vi "Read DTCs.vi"(8 "error in (no error)":errorcluster, 11 "Node Ptr":T2 format="%.0x") -> (0 "error out":errorcluster)   [LabVIEW 2024, in "Diagnostics Addon System Explorer.lvlib"]
uses:
  Diagnostics Addon System Explorer.lvlib
  <vilib>/NI VeriStand/Custom Device API/Custom Device Item Ref.ctl
  Types/FG.Action.ctl
  Addon Shared/Types/DTC.Settings.ctl
  Addon Shared/Types/DTC.Descriptor.ctl
  <vilib>/NI VeriStand/Custom Device API/Custom Device Channel.ctl
  <vilib>/NI VeriStand/Custom Device API/Custom Device Channel Type.ctl
  Addon Shared/SubVIs/Constants.vi
  <vilib>/NI VeriStand/Custom Device Tools/Custom Device Utility Library/NI VeriStand - Search for All Items by GUID.vi
  <vilib>/NI/NI VeriStand Advanced SysDef API/SysDef API/SysDef.Property.Set.vi
  <vilib>/NI/NI VeriStand Advanced SysDef API/_SubVIs/SysDef.Property.Set.I32.vi
  <vilib>/NI/NI VeriStand Advanced SysDef API/_SubVIs/SysDef.Property.Set.U32.vi
  <vilib>/NI/NI VeriStand Advanced SysDef API/_SubVIs/SysDef.Property.Set.DBL.Array.vi
  <vilib>/NI/NI VeriStand Advanced SysDef API/_SubVIs/SysDef.Property.Set.String.Array.vi
  <vilib>/NI VeriStand/Custom Device API/NI VeriStand - Get Item Property.vi
  <vilib>/NI VeriStand/Custom Device API/Get Item Property (I32).vi
  <vilib>/NI VeriStand/Custom Device API/Get Item Property (U32).vi
  <vilib>/NI VeriStand/Custom Device API/Get Item Property (Double Array).vi
  <vilib>/NI VeriStand/Custom Device API/Get Item Property (String Array).vi
  <vilib>/NI VeriStand/Custom Device Tools/Custom Device Utility Library/NI VeriStand - Search for Item by GUID.vi
  <vilib>/NI VeriStand/Custom Device API/Custom Device API.lvlib
  Addon Shared/Diagnostics Addon Shared.lvlib
  <vilib>/NI VeriStand/Custom Device Tools/Custom Device Utility Library/Custom Device Utility Library.lvlib
panel:
  in  "Clear":bool
  in  "Code Tabs":T1(tab)
  in  "DTC Byte Length":i32=2
  in  "Status Byte Length":i32=1
  in  "Failure Byte Length":i32=1
  in  "Byte Order":enum16{"Motorola", "Intel"}(ring)
  in  "DTC Codes":i32(listbox)
  in  "Status Codes":i32(listbox)
  in  "Import":bool
  in  "Apply":bool
  in  "Number of DTCs":u32=10 min=1 step=1
  in  "Header 2":cluster{"Section Name":string}={"Section Name"="Number of DTCs to Acquire"}
  in  "Description":string
  out "Name":string
  in  "SHDocVw.IWebBrowser":refnum<k7>(container)
  in  "Header":cluster{"Section Name":string}={"Section Name"="DTC Settings"}
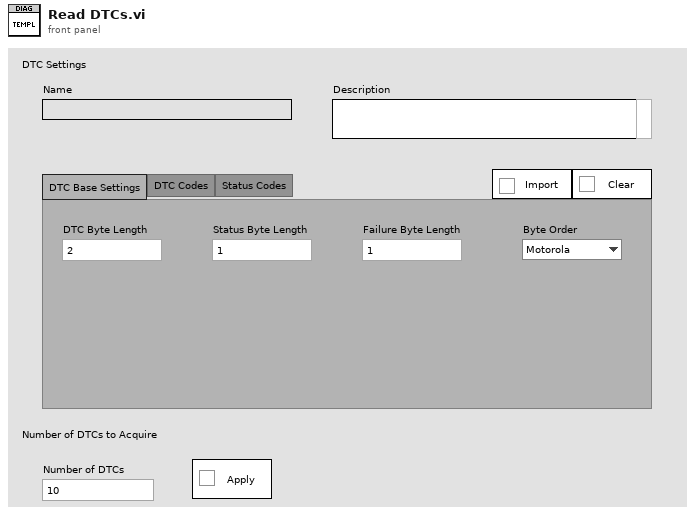
[diagram p1: front panel]
types:
  T1 = enum32{"DTC Base Settings", "DTC Codes", "Status Codes"}
  T2 = typedef "Custom Device API.lvlib/Custom Device Item Ref.ctl" = u64
  T3 = typedef "Diagnostics Addon Shared.lvlib/DTC.Settings.ctl" = cluster{"Descriptor":T4, "Value.Code":dbl[], "Value.String":string[], "Value.J2012String":string[], "Status.Code":dbl[], "Status.String":string[]}
  T4 = typedef "Diagnostics Addon Shared.lvlib/DTC.Descriptor.ctl" = cluster{"DTC Byte Length":i32, "Status Byte Length":i32, "Add Data Byte Length":i32, "Byte Order":enum16{"Motorola", "Intel"}}
  T5 = typedef "Diagnostics Addon System Explorer.lvlib/FG.Action.ctl" = enum16{"Get", "Set"}
  T6 = typedef "Custom Device API.lvlib/Custom Device Item Info.ctl" = cluster{"Name":string, "Is Channel":bool, "GUID":string, "Is Waveform":bool}
  T7 = typedef "Custom Device API.lvlib/Custom Device Channel.ctl" = cluster{"Type":T8, "Units":string, "Default Value":dbl, "Faultable":bool, "Scalable":bool}
  T8 = typedef "Custom Device API.lvlib/Custom Device Channel Type.ctl" = enum16{"Input", "Output"}
  T9 = typedef "Custom Device API.lvlib/Custom Device Commands.ctl" = enum16{"Default", "Item renamed", "Shutdown", "Dynamic button pressed"}
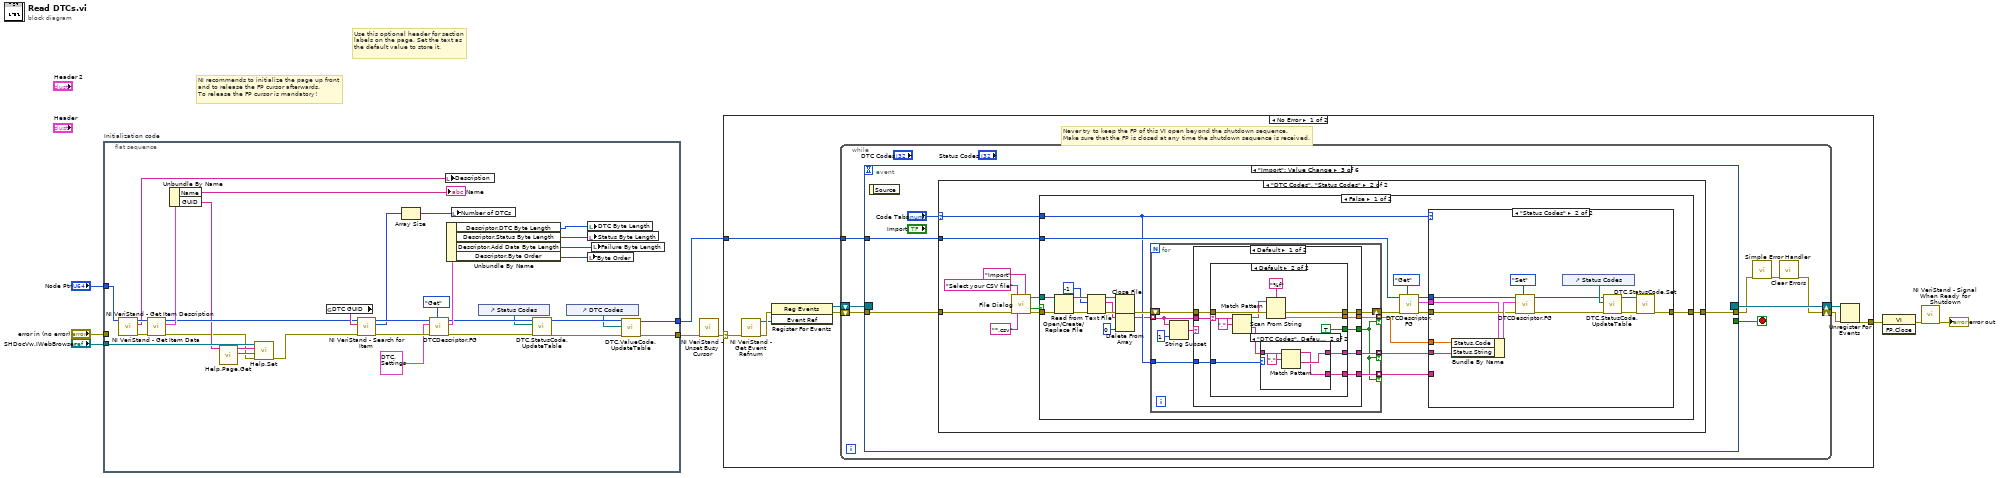
[diagram p0: block diagram]
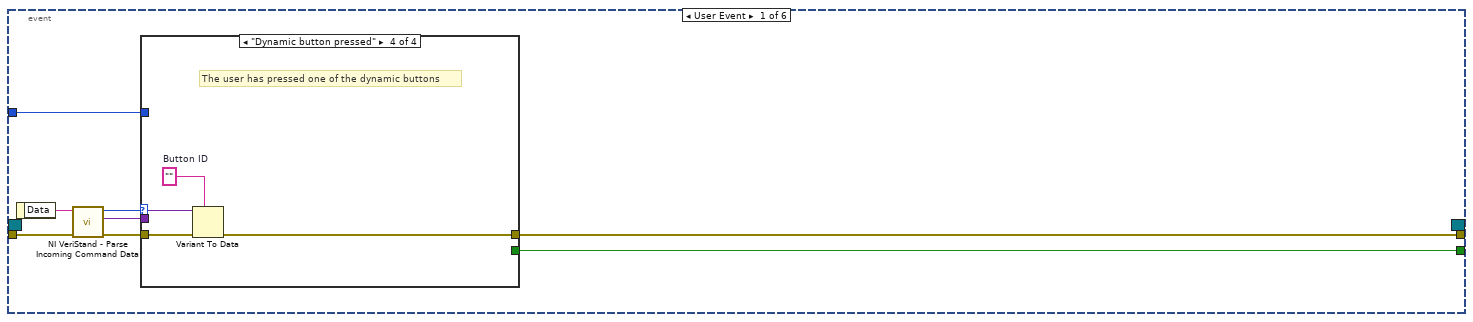
[diagram p2: hidden frame]
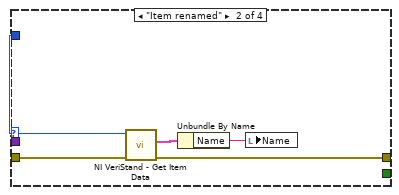
[diagram p4: hidden frame]
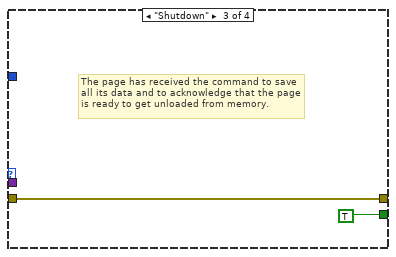
[diagram p5: hidden frame]
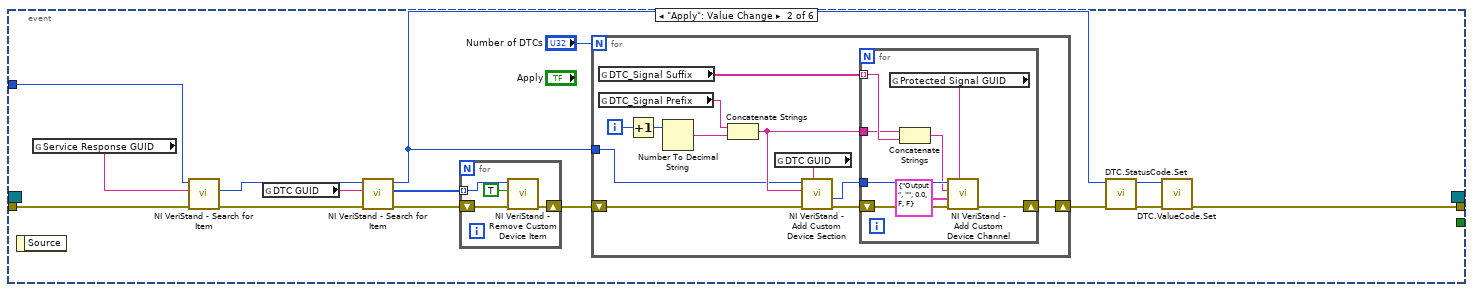
[diagram p6: hidden frame]
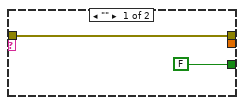
[diagram p8: hidden frame]
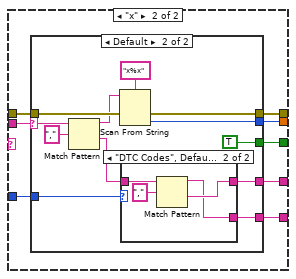
[diagram p10: hidden frame]
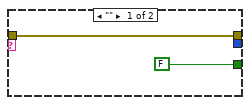
[diagram p11: hidden frame]
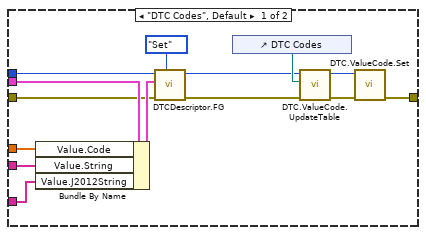
[diagram p13: hidden frame]
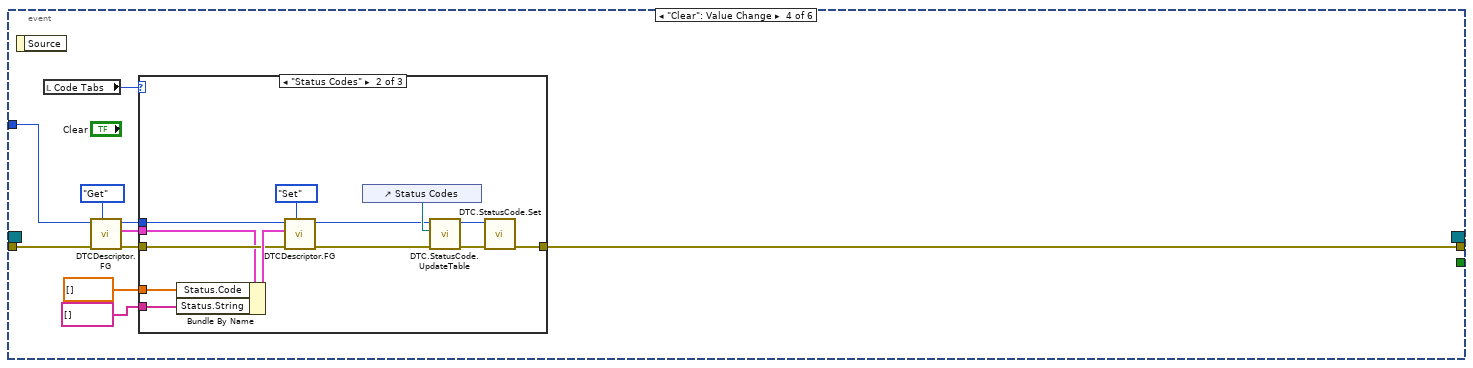
[diagram p15: hidden frame]
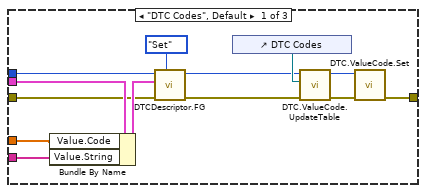
[diagram p16: hidden frame]
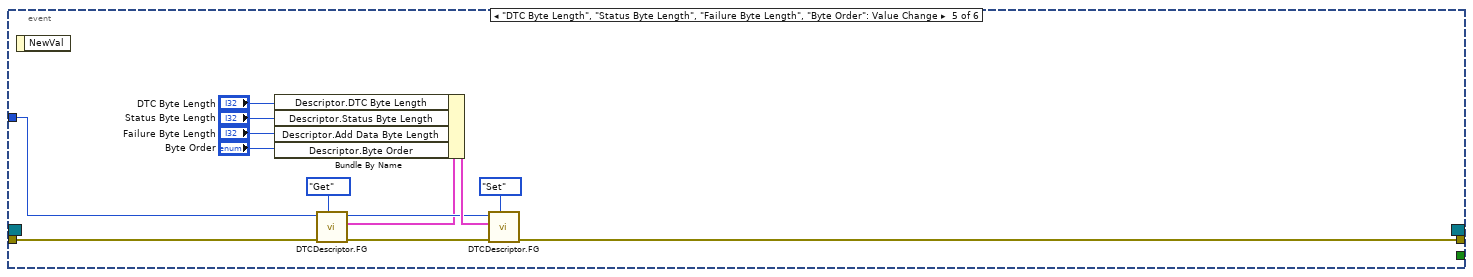
[diagram p18: hidden frame]
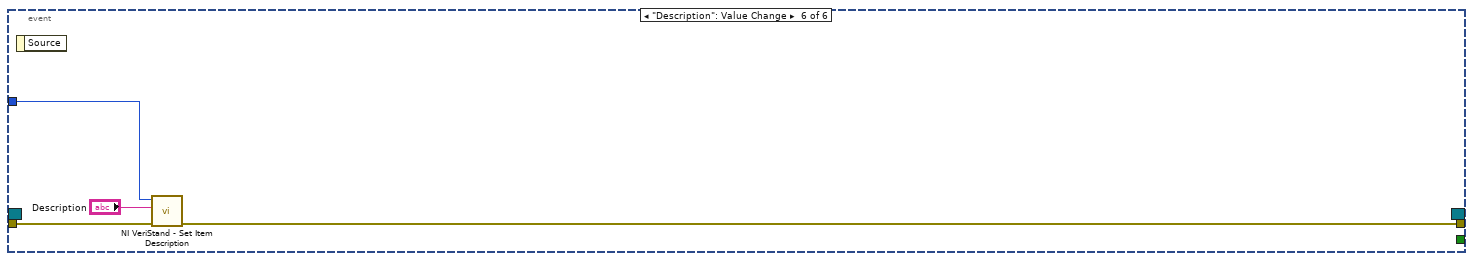
[diagram p19: hidden frame]
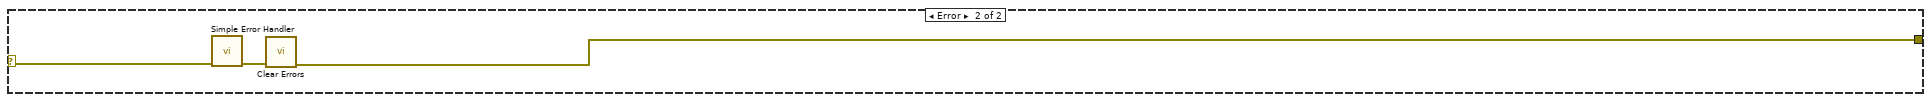
[diagram p20: hidden frame]
diagram:
  # "Use this optional header for section labels on the page. Set the text as the default value to store it."
  # "NI recommends to initialize the page up front\nand to release the FP cursor afterwards.\nTo release the FP cursor is mandatory!"
  n1 = flat-sequence "Initialization code" {
    tunnel: "error in (no error)" -> [_]
    tunnel: "Node Ptr" -> [w15]
    tunnel: [w21] -> w5
    tunnel: [w19] -> w2
    tunnel: "SHDocVw.IWebBrowser" -> [w38]
    frame #0 {
      n2 = call <vilib>:"NI VeriStand - Get Item Description.vi"("Item Ref in"=w15) -> ("error out"=w40:errorcluster, "Description"=w41:string, "Item Ref out"=w42:T2)  [unwired: 1 in, 7 out]
      n3 = call <vilib>:"NI VeriStand - Get Item Data.vi"("error in (no error)"=w40, "Item Ref in"=w42) -> ("error out"=w11:errorcluster, "Item Info"=w39:T6, "Item Ref out"=w29:T2)  [unwired: 7 out]
      n4 = Unbundle By Name(w39) -> ("Name"=→"Name":string, "GUID"=w12:string)
      n5 = call "Help.Page.Get.vi"("GUID"=w12) -> ("HTML File"=w13:string, "Main CHM File"=w14:string)  [unwired: 9 in]
      n6 = call "Help.Set.vi"("error in (no error)"=w11, "HTML File"=w13, "Main CHM File"=w14, "SHDocVw.IWebBrowser2"=w38) -> ("error out"=w10:errorcluster)  [unwired: 7 in]
      n7 = global read "Constants.vi" "DTC GUID"() -> (w30:string)
      n8 = call-poly <vilib>:"NI VeriStand - Search for Item.vi"("error in"=w10, "Item GUID"=w30, "Section Ref in"=w29) -> ("error out"=w27:errorcluster, "Item Refs"=w26:T2[], "Section Ref out"=w28:T2)  [unwired: 5 in, 1 out]
      n9 = Array Size(array=w26) -> (size(s)=w25:i32)
      n10 = call "DTCDescriptor.FG.vi"("Action"=FG.Action."Get", "error in (no error)"=w27, "DTC"=T3 {"Descriptor"={"DTC Byte Length"=2, "Status Byte Length"=1, "Add Data Byte Length"=1, "Byte Order"=enum."Motorola"}, "Value.Code"=[], "Value.String"=[], "Value.J2012String"=[], "Status.Code"=[], "Status.String"=[]}, "Device Item Ref in"=w28) -> ("error out"=w22:errorcluster, "DTC descriptor"=w37:T3, "Device Item Ref out"=w20:T2)  [unwired: 5 in]
      n11 = local write "Description"(w41) -> ()
      n12 = Unbundle By Name(w37) -> ("Descriptor.DTC Byte Length"=w36:i32, "Descriptor.Status Byte Length"=w33:i32, "Descriptor.Add Data Byte Length"=w34:i32, "Descriptor.Byte Order"=w35:enum16{"Motorola", "Intel"})
      n13 = local write "Number of DTCs"(w25) -> ()
      n14 = control-ref of="Status Codes"() -> (w17:refnum<vi>)
      n15 = call "DTC.StatusCode.UpdateTable.vi"("error in (no error)"=w22, "Status Codes"=w17, "Device Item Ref in"=w20) -> ("error out"=w23:errorcluster, "Device Item Ref out"=w24:T2)  [unwired: 7 in]
      n16 = control-ref of="DTC Codes"() -> (w18:refnum<vi>)
      n17 = local write "Byte Order"(w35) -> ()
      n18 = local write "DTC Byte Length"(w36) -> ()
      n19 = local write "Status Byte Length"(w33) -> ()
      n20 = local write "Failure Byte Length"(w34) -> ()
      n21 = call "DTC.ValueCode.UpdateTable.vi"("error in (no error)"=w23, "DTC Codes"=w18, "Device Item Ref in"=w24) -> ("error out"=w21:errorcluster, "Device Item Ref out"=w19:T2)  [unwired: 7 in]
    }
  }
  n22 = call <vilib>:"NI VeriStand - Unset Busy Cursor.vi"("error in (no error)"=w5) -> ("error out"=w4:errorcluster)  [unwired: 10 out]
  n23 = case shown="No Error" w4 {
    selector: w4 -> [w43 w302]
    tunnel: [w48 w300] -> w9
    tunnel: w2 -> [w44 _]
    frame No Error {
      # "Never try to keep the FP of this VI open beyond the shutdown sequence.\nMake sure that the FP is closed at any time the shutdown sequence is received."
      n24 = call <vilib>:"NI VeriStand - Get Event Refnum.vi"("error in (no error)"=w43) -> ("error out"=w51:errorcluster, "Event Ref"=w47:refnum<user-event>)  [unwired: 9 out]
      n25 = register-events(error in=w51, w47) -> (reference out=w45:refnum<event-registration>, error out=w46:errorcluster)  [unwired: 1 in]
      n26 = while {
        tunnel: w44 -> [w55]
        shift-right: [w52] -> w49
        shift-left: w46 -> [w58]
        shift-right: [w59] -> w50
        shift-left: w45 -> [w57]
        stop <- w56 stop-if-true
        n27 = event shown="[2] \"Import\": Value Change" {
          selector: w57 -> [_ _ _ _ _ _]
          dyn-events: [_ _ _ _ _ _] -> w59
          timeout: _ -> [_ _ _ _ _ _]
          tunnel: w58 -> [w67 w84 w120 w249 w290 w298]
          tunnel: [w63 _ _ _ _ _] -> w56
          tunnel: [w62 w86 w121 w255 w289 w297] -> w54
          tunnel: w55 -> [w61 w81 w122 w256 w286 w299]
          event User Event {
            n28 = event-data() -> ("Data"=w66:string)  [unwired: 1 out]
            n29 = call <vilib>:"NI VeriStand - Parse Incoming Command Data.vi"("error in (no error)"=w67, "Incoming data"=w66) -> ("error out"=w65:errorcluster, "Outgoing data"=w60:variant, "Action"=w64:T9)  [unwired: 7 out]
            n30 = case shown="\"Dynamic button pressed\"" w64 {
              tunnel: w65 -> [w68 w73 w74 w79]
              tunnel: [_ _ TRUE _] -> w63
              tunnel: [w68 w70 w74 w76] -> w62
              tunnel: w61 -> [_ w72 _ _]
              tunnel: w60 -> [_ _ _ w78]
              frame "Default", Default {
              }
              frame "Item renamed" {
                n31 = call <vilib>:"NI VeriStand - Get Item Data.vi"("error in (no error)"=w73, "Item Ref in"=w72) -> ("error out"=w70:errorcluster, "Item Info"=w71:T6)  [unwired: 8 out]
                n32 = Unbundle By Name(w71) -> ("Name"=w69:string)
                n33 = local write "Name"(w69) -> ()
              }
              frame "Shutdown" {
                # "The page has received the command to save all its data and to acknowledge that the page is ready to get unloaded from memory."
              }
              frame "Dynamic button pressed" {
                w77 = ""  # Button ID
                # "The user has pressed one of the dynamic buttons"
                n34 = Variant To Data(error in=w79, type=w77, Variant=w78) -> (error out=w76:errorcluster)  [unwired: 1 out]
              }
            }
          }
          event "Apply": Value Change {
            n35 = event-data() -> ()  [unwired: 2 out]
            n36 = global read "Constants.vi" "Service Response GUID"() -> (w80:string)
            n37 = call-poly <vilib>:"NI VeriStand - Search for Item.vi"("error in"=w84, "Item GUID"=w80, "Section Ref in"=w81) -> ("error out"=w83:errorcluster, "Item Ref"=w82:T2)  [unwired: 5 in, 2 out]
            n38 = global read "Constants.vi" "DTC GUID"() -> (w93:string)
            n39 = call-poly <vilib>:"NI VeriStand - Search for Item.vi"("error in"=w83, "Item GUID"=w93, "Section Ref in"=w82) -> ("error out"=w92:errorcluster, "Item Refs"=w90:T2[], "Section Ref out"=w85:T2)  [unwired: 5 in, 1 out]
            n40 = for {
              shift-right: [w97] -> w91
              shift-left: w92 -> [w98]
              tunnel: w90 -> [w96] mode=indexing
              n41 = call <vilib>:"NI VeriStand - Remove Custom Device Item.vi"("error in (no error)"=w98, "Force Delete (F)"=TRUE, "Item Ref in"=w96) -> ("error out"=w97:errorcluster)  [unwired: 7 in, 1 out]
            }
            n42 = for {
              N: "Number of DTCs" -> [_]
              shift-right: [w110] -> w87
              shift-left: w91 -> [w105]
              tunnel: w85 -> [w99]
              i -> [w109]
              n43 = global read "Constants.vi" "DTC_Signal Suffix"() -> (w102:string[])
              n44 = global read "Constants.vi" "DTC_Signal Prefix"() -> (w101:string)
              n45 = Increment(x=w109) -> (x+1=w108:i32)
              n46 = Number To Decimal String(number=w108) -> (decimal integer string=w107:string)  [unwired: 1 in]
              n47 = Concatenate Strings(w101, w107) -> (w103:string)
              n48 = global read "Constants.vi" "DTC GUID"() -> (w100:string)
              n49 = call <vilib>:"NI VeriStand - Add Custom Device Section.vi"("GUID (Default Section)"=w100, "error in (no error)"=w105, "Section Name"=w103, "Parent Ref in"=w99) -> ("error out"=w104:errorcluster, "Section Ptr"=w106:T2)  [unwired: 4 in, 2 out]
              n50 = for {
                tunnel: w106 -> [w116]
                tunnel: w103 -> [w113]
                tunnel: w102 -> [w114] mode=indexing
                shift-right: [w118] -> w110
                shift-left: w104 -> [w115]
                n51 = global read "Constants.vi" "Protected Signal GUID"() -> (w111:string)
                n52 = Concatenate Strings(w113, w114) -> (w112:string)
                n53 = call <vilib>:"NI VeriStand - Add Custom Device Channel.vi"("GUID (Default Channel)"=w111, "error in (no error)"=w115, "Channel"=T7 {"Type"=enum."Output", "Units"="", "Default Value"=0.0, "Faultable"=FALSE, "Scalable"=FALSE}, "Channel Name"=w112, "Parent Ref in"=w116) -> ("error out"=w118:errorcluster)  [unwired: 3 in, 3 out]
              }
            }
            n54 = call "DTC.StatusCode.Set.vi"("error in"=w87, "Section Ref in"=w85) -> ("error out"=w89:errorcluster, "Section Ref out"=w88:T2)  [unwired: 8 in]
            n55 = call "DTC.ValueCode.Set.vi"("error in"=w89, "Section Ref in"=w88) -> ("error out"=w86:errorcluster)  [unwired: 8 in, 1 out]
          }
          event "Import": Value Change {
            n56 = event-data() -> ()  [unwired: 2 out]
            n57 = case shown="\"DTC Codes\", \"Status Codes\"" "Code Tabs" {
              selector: "Code Tabs" -> [_ w124]
              tunnel: w122 -> [_ w133]
              tunnel: [w123 w132] -> w121
              tunnel: w120 -> [w123 w128]
              frame "DTC Base Settings", Default {
              }
              frame "DTC Codes", "Status Codes" {
                n58 = call "File Dialog"("prompt"="Select your CSV file", "button label"="Import", "error in"=w128, "pattern (all files)"="*.csv") -> ("selected path"=w125:path, "cancelled"=w126:bool, "error out"=w127:errorcluster)  [unwired: 8 in, 1 out]
                n59 = case shown="False" w126 {
                  tunnel: w124 -> [w138 _]
                  tunnel: w133 -> [w154 _]
                  tunnel: [w150 _] -> w132
                  tunnel: w127 -> [w147 _]
                  tunnel: w125 -> [w144 _]
                  frame False {
                    n60 = Open/Create/Replace File(file path (use dialog)=w144, error in=w147) -> (refnum out=w145:refnum<file>, error out=w149:errorcluster)  [unwired: 4 in, 1 out]
                    n61 = Read from Text File(file (use dialog)=w145, count=-1, error in=w149) -> (refnum out=w146:refnum<file>, text=w135:string[], error out=w148:errorcluster)  [unwired: 1 in, 1 out]
                    n62 = Close File(refnum=w146, error in=w148) -> (error out=w142:errorcluster)  [unwired: 1 out]
                    n63 = Delete From Array(array=w135, index=0) -> (array with subset deleted=w136:string[])  [unwired: 1 in, 1 out]
                    n64 = for {
                      tunnel: w136 -> [w161] mode=indexing
                      shift-right: [w164] -> w141
                      shift-left: w142 -> [w165]
                      tunnel: [w163] -> w140 mode=indexing if=w156
                      tunnel: [w162] -> w139 mode=indexing if=w156
                      tunnel: w138 -> [w158]
                      tunnel: [w157] -> w137 mode=indexing if=w156
                      n65 = String Subset(string=w161, length (rest)=1 ("length (rest)")) -> (substring=w159:string)  [unwired: 1 in]
                      n66 = case shown="Default" w159 {
                        tunnel: w165 -> [w173 w200]
                        tunnel: [w172 w199] -> w164
                        tunnel: [w171 w198] -> w163
                        tunnel: [w170 w197] -> w162
                        tunnel: [w169 w196] -> w156
                        tunnel: w161 -> [w168 w195]
                        tunnel: w158 -> [w167 w194]
                        tunnel: [w166 w193] -> w157
                        frame Default {
                          n67 = case shown="Default" w168 {
                            selector: w168 -> [_ w181]
                            tunnel: w173 -> [w175 w186]
                            tunnel: [w175 w185] -> w172
                            tunnel: [_ w184] -> w171
                            tunnel: [_ w178] -> w170
                            tunnel: [FALSE TRUE] -> w169
                            tunnel: w167 -> [_ w176]
                            tunnel: [_ w177] -> w166
                            frame "" {
                            }
                            frame Default {
                              n68 = Match Pattern(string=w181, regular expression=",") -> (before substring=w180:string, after substring=w179:string)  [unwired: 1 in, 2 out]
                              n69 = case shown="\"DTC Codes\", Default" w176 {
                                tunnel: w179 -> [w188 w191]
                                tunnel: [w188 w190] -> w178
                                tunnel: [_ w189] -> w177
                                frame "Status Codes" {
                                }
                                frame "DTC Codes", Default {
                                n70 = Match Pattern(string=w191, regular expression=",") -> (before substring=w189:string, after substring=w190:string)  [unwired: 1 in, 2 out]
                                }
                              }
                              n71 = Scan From String(format string="%f", input string=w180, error in=w186) -> (error out=w185:errorcluster, output 1=w184:dbl)  [unwired: 2 in, 2 out]
                            }
                          }
                        }
                        frame "x" {
                          n72 = case shown="Default" w195 {
                            selector: w195 -> [_ w208]
                            tunnel: w200 -> [w202 w213]
                            tunnel: [w202 w212] -> w199
                            tunnel: [_ w211] -> w198
                            tunnel: [_ w204] -> w197
                            tunnel: [FALSE TRUE] -> w196
                            tunnel: w194 -> [_ w206]
                            tunnel: [_ w203] -> w193
                            frame "" {
                            }
                            frame Default {
                              n73 = Match Pattern(string=w208, regular expression=",") -> (before substring=w207:string, after substring=w205:string)  [unwired: 1 in, 2 out]
                              n74 = Scan From String(format string="x%x", input string=w207, error in=w213) -> (error out=w212:errorcluster, output 1=w211:u32)  [unwired: 2 in, 2 out]
                              n75 = case shown="\"DTC Codes\", Default" w206 {
                                tunnel: w205 -> [w215 w218]
                                tunnel: [w215 w217] -> w204
                                tunnel: [_ w216] -> w203
                                frame "Status Codes" {
                                }
                                frame "DTC Codes", Default {
                                n76 = Match Pattern(string=w218, regular expression=",") -> (before substring=w216:string, after substring=w217:string)  [unwired: 1 in, 2 out]
                                }
                              }
                            }
                          }
                        }
                      }
                    }
                    n77 = call "DTCDescriptor.FG.vi"("Action"=FG.Action."Get", "error in (no error)"=w141, "Device Item Ref in"=w154) -> ("error out"=w153:errorcluster, "DTC descriptor"=w151:T3, "Device Item Ref out"=w152:T2)  [unwired: 6 in]
                    n78 = case shown="\"Status Codes\"" w138 {
                      tunnel: w153 -> [w227 w241]
                      tunnel: w152 -> [w226 w239]
                      tunnel: w151 -> [w229 w240]
                      tunnel: [w223 w236] -> w150
                      tunnel: w140 -> [w222 w235]
                      tunnel: w139 -> [w221 w234]
                      tunnel: w137 -> [w220 _]
                      frame "DTC Codes", Default {
                        n79 = Bundle By Name(cluster=w229, "Value.Code"=w222, "Value.String"=w221, "Value.J2012String"=w220) -> (w228:T3)
                        n80 = call "DTCDescriptor.FG.vi"("Action"=FG.Action."Set", "error in (no error)"=w227, "DTC"=w228, "Device Item Ref in"=w226) -> ("error out"=w225:errorcluster, "Device Item Ref out"=w224:T2)  [unwired: 5 in, 1 out]
                        n81 = control-ref of="DTC Codes"() -> (w233:refnum<vi>)
                        n82 = call "DTC.ValueCode.UpdateTable.vi"("error in (no error)"=w225, "DTC Codes"=w233, "Device Item Ref in"=w224) -> ("error out"=w232:errorcluster, "Device Item Ref out"=w231:T2)  [unwired: 7 in]
                        n83 = call "DTC.ValueCode.Set.vi"("error in"=w232, "Section Ref in"=w231) -> ("error out"=w223:errorcluster)  [unwired: 8 in, 1 out]
                      }
                      frame "Status Codes" {
                        n84 = Bundle By Name(cluster=w240, "Status.Code"=w235, "Status.String"=w234) -> (w242:T3)
                        n85 = call "DTCDescriptor.FG.vi"("Action"=FG.Action."Set", "error in (no error)"=w241, "DTC"=w242, "Device Item Ref in"=w239) -> ("error out"=w238:errorcluster, "Device Item Ref out"=w237:T2)  [unwired: 5 in, 1 out]
                        n86 = control-ref of="Status Codes"() -> (w246:refnum<vi>)
                        n87 = call "DTC.StatusCode.UpdateTable.vi"("error in (no error)"=w238, "Status Codes"=w246, "Device Item Ref in"=w237) -> ("error out"=w244:errorcluster, "Device Item Ref out"=w245:T2)  [unwired: 7 in]
                        n88 = call "DTC.StatusCode.Set.vi"("error in"=w244, "Section Ref in"=w245) -> ("error out"=w236:errorcluster)  [unwired: 8 in, 1 out]
                      }
                    }
                  }
                  frame True {
                  }
                }
              }
            }
          }
          event "Clear": Value Change {
            n89 = event-data() -> ()  [unwired: 2 out]
            n90 = local read "Code Tabs"() -> (w254:T1)
            n91 = call "DTCDescriptor.FG.vi"("Action"=FG.Action."Get", "error in (no error)"=w249, "Device Item Ref in"=w256) -> ("error out"=w252:errorcluster, "DTC descriptor"=w250:T3, "Device Item Ref out"=w251:T2)  [unwired: 6 in]
            n92 = case shown="\"Status Codes\"" w254 {
              tunnel: w252 -> [w263 w277 w283]
              tunnel: w251 -> [w262 w275 _]
              tunnel: w250 -> [w265 w276 _]
              tunnel: [w259 w272 w283] -> w255
              tunnel: dbl[] [] -> [w258 w271 _]
              tunnel: string[] [] -> [w257 w270 _]
              frame "DTC Codes", Default {
                n93 = Bundle By Name(cluster=w265, "Value.Code"=w258, "Value.String"=w257) -> (w264:T3)
                n94 = call "DTCDescriptor.FG.vi"("Action"=FG.Action."Set", "error in (no error)"=w263, "DTC"=w264, "Device Item Ref in"=w262) -> ("error out"=w261:errorcluster, "Device Item Ref out"=w260:T2)  [unwired: 5 in, 1 out]
                n95 = control-ref of="DTC Codes"() -> (w269:refnum<vi>)
                n96 = call "DTC.ValueCode.UpdateTable.vi"("error in (no error)"=w261, "DTC Codes"=w269, "Device Item Ref in"=w260) -> ("error out"=w268:errorcluster, "Device Item Ref out"=w267:T2)  [unwired: 7 in]
                n97 = call "DTC.ValueCode.Set.vi"("error in"=w268, "Section Ref in"=w267) -> ("error out"=w259:errorcluster)  [unwired: 8 in, 1 out]
              }
              frame "Status Codes" {
                n98 = Bundle By Name(cluster=w276, "Status.Code"=w271, "Status.String"=w270) -> (w278:T3)
                n99 = call "DTCDescriptor.FG.vi"("Action"=FG.Action."Set", "error in (no error)"=w277, "DTC"=w278, "Device Item Ref in"=w275) -> ("error out"=w274:errorcluster, "Device Item Ref out"=w273:T2)  [unwired: 5 in, 1 out]
                n100 = control-ref of="Status Codes"() -> (w282:refnum<vi>)
                n101 = call "DTC.StatusCode.UpdateTable.vi"("error in (no error)"=w274, "Status Codes"=w282, "Device Item Ref in"=w273) -> ("error out"=w280:errorcluster, "Device Item Ref out"=w281:T2)  [unwired: 7 in]
                n102 = call "DTC.StatusCode.Set.vi"("error in"=w280, "Section Ref in"=w281) -> ("error out"=w272:errorcluster)  [unwired: 8 in, 1 out]
              }
              frame "DTC Base Settings" {
              }
            }
          }
          event "DTC Byte Length", "Status Byte Length", "Failure Byte Length", "Byte Order": Value Change {
            n103 = event-data() -> ()  [unwired: 2 out]
            n104 = call "DTCDescriptor.FG.vi"("Action"=FG.Action."Get", "Device Item Ref in"=w286) -> ("DTC descriptor"=w284:T3, "Device Item Ref out"=w285:T2)  [unwired: 7 in, 1 out]
            n105 = Bundle By Name(cluster=w284, "Descriptor.DTC Byte Length"="DTC Byte Length", "Descriptor.Status Byte Length"="Status Byte Length", "Descriptor.Add Data Byte Length"="Failure Byte Length", "Descriptor.Byte Order"="Byte Order") -> (w288:T3)
            n106 = call "DTCDescriptor.FG.vi"("Action"=FG.Action."Set", "error in (no error)"=w290, "DTC"=w288, "Device Item Ref in"=w285) -> ("error out"=w289:errorcluster)  [unwired: 5 in, 2 out]
          }
          event "Description": Value Change {
            n107 = event-data() -> ()  [unwired: 2 out]
            n108 = call <vilib>:"NI VeriStand - Set Item Description.vi"("error in (no error)"=w298, "Description"="Description", "Item Ref in"=w299) -> ("error out"=w297:errorcluster)  [unwired: 8 out]
          }
        }
        n109 = call <vilib>:"Simple Error Handler.vi"("error in (no error)"=w54) -> ("error out"=w53:errorcluster)  [unwired: 1 in, 7 out]
        n110 = call <vilib>:"Clear Errors.vi"("error in (no error)"=w53) -> ("error out"=w52:errorcluster)  [unwired: 1 in, 5 out]
      }
      n111 = Unregister For Events(event registration refnum=w50, error in=w49) -> (error out=w48:errorcluster)
    }
    frame Error {
      n112 = call <vilib>:"Simple Error Handler.vi"("error in (no error)"=w302) -> ("error out"=w301:errorcluster)  [unwired: 1 in, 7 out]
      n113 = call <vilib>:"Clear Errors.vi"("error in (no error)"=w301) -> ("error out"=w300:errorcluster)  [unwired: 1 in, 5 out]
    }
  }
  n114 = invoke class="VI" method="FP.Close"(error in=w9) -> (error out=w8:errorcluster)  [unwired: 2 in, 2 out]
  n115 = call <vilib>:"NI VeriStand - Signal When Ready for Shutdown.vi"("error in (no error)"=w8) -> ("error out"=→"error out":errorcluster)  [unwired: 10 out]
